vi "slscsl_connect.vi"(8 "error in (no error)":errorcluster, 10 "connectionList":string, 11 "slscsl in":refnum<class "slscsl.lvclass">) -> (0 "error out":errorcluster, 2 "switchActionsArray":T1 {"RelayAction" items=["CloseRelay"=21, "OpenRelay"=20]}, 3 "slscsl out":refnum<class "slscsl.lvclass">)   [LabVIEW 2015, in "SLSC Switch.lvlib" / "slscsl.lvclass"]
uses:
  slscsl.lvclass
  SwitchActionsArray.ctl
  SwitchAction.ctl
  RelayAction.ctl
  slscsl.lvclass/slscsl.ctl
  slscsl32.dll
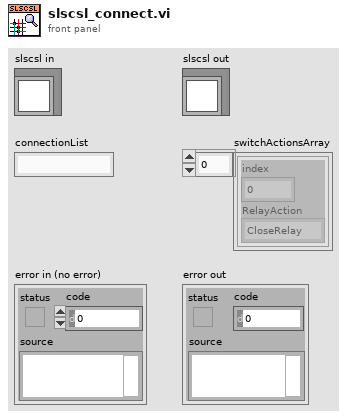
[diagram p1: front panel]
types:
  T1 = typedef "SLSC Switch.lvlib/slscsl.lvclass/SwitchActionsArray.ctl" = T2[]
  T2 = typedef "SLSC Switch.lvlib/slscsl.lvclass/SwitchAction.ctl" = cluster{"index":i32, "RelayAction":T3}
  T3 = typedef "SLSC Switch.lvlib/slscsl.lvclass/RelayAction.ctl" = u32
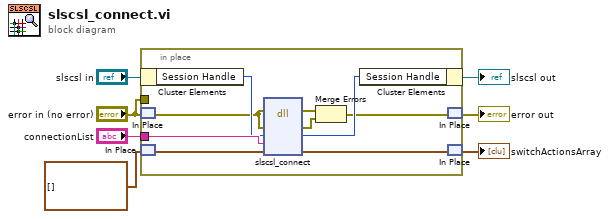
[diagram p0: block diagram]
diagram:
  n1 = in-place {
    in-place-border: "error in (no error)" -> [_]
    in-place-border: "connectionList" -> [w13]
    n2 = in-place-cluster #1("slscsl in") -> ("Session Handle"=w12:u64)
    n3 = in-place-match #2("error in (no error)") -> (w11:errorcluster)
    n4 = in-place-match #3(T1 [] ("SwitchActionList")) -> (w9:T1)
    n5 = dll-call lib="slscsl*.dll" fn="slscsl_connect"(error in=w11, "errorCluster"=w11, "sessionHandle"=w12, "connectionList"=w13, "switchActionsArray"=w9) -> (error out=w16:errorcluster, "errorCluster"=w15:errorcluster, "sessionHandle"=w14:u64, "switchActionsArray"=w8:T1)  [unwired: 4 in, 1 out]
    n6 = Merge Errors(w16, w15) -> (w10:errorcluster)
    n7 = in-place-cluster #1("Session Handle"=w14) -> (→"slscsl out":refnum<class "slscsl.lvclass">)
    n8 = in-place-match #2(w10) -> (→"error out":errorcluster)
    n9 = in-place-match #3(w8) -> (→"switchActionsArray":T1)
  }
